vi "Create HDF5 chunked dataset (1D).vi"(5 "block size":i32, 6 "compression":i32, 8 "error in (no error)":errorcluster, 9 "data type":variant, 10 "name":string="stuff", 11 "ref in":T1 format="%.0x") -> (0 "error out":errorcluster, 3 "dset out":i32)   [LabVIEW 2013]
uses:
  <vilib>/addons/h5labview2/base/hid_t.ctl
  <vilib>/addons/h5labview2/dataset/H5D.lvlib
  <vilib>/addons/h5labview2/space/H5S.lvlib
  <vilib>/addons/h5labview2/props/H5P.lvlib
  <vilib>/addons/h5labview2/type/H5T.lvlib
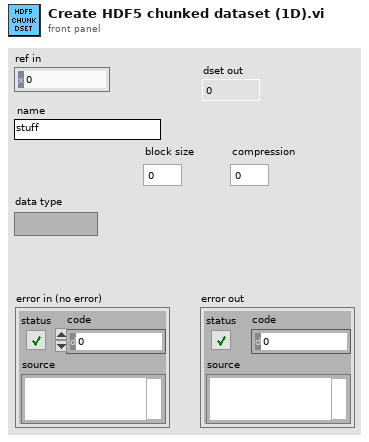
[diagram p1: front panel]
types:
  T1 = typedef "hid_t.ctl" = i32
  T2 = enum16{"H5P_ROOT", "H5P_OBJECT_CREATE", "H5P_FILE_CREATE", "H5P_FILE_ACCESS", "H5P_DATASET_CREATE", "H5P_DATASET_ACCESS", "H5P_DATASET_XFER", "H5P_FILE_MOUNT", "H5P_GROUP_CREATE", "H5P_GROUP_ACCESS", "H5P_DATATYPE_CREATE", "H5P_DATATYPE_ACCESS", "H5P_STRING_CREATE", "H5P_ATTRIBUTE_CREATE", "H5P_OBJECT_COPY", "H5P_LINK_CREATE", "H5P_LINK_ACCESS"}
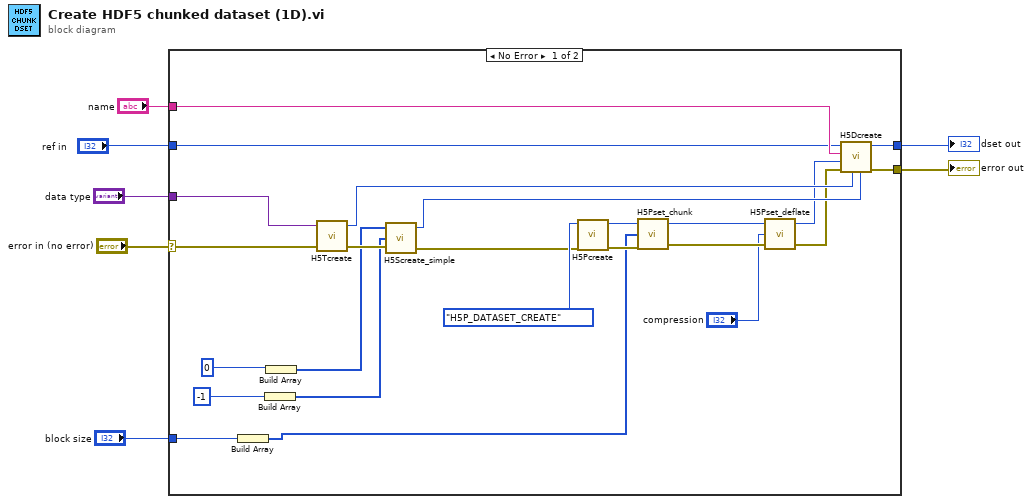
[diagram p0: block diagram]
diagram:
  n1 = case shown="No Error" "error in (no error)" {
    selector: "error in (no error)" -> [w12 w32]
    tunnel: [w31 w32] -> w7
    tunnel: [w30 _] -> w6
    tunnel: "name" -> [w24 _]
    tunnel: "ref in" -> [w23 _]
    tunnel: "data type" -> [w22 _]
    tunnel: "block size" -> [w21 _]
    frame No Error {
      n2 = Build Array(w21) -> (w20:i32[])
      n3 = Build Array(-1 ("element")) -> (w8:i32[])
      n4 = Build Array(0 ("element")) -> (w10:i32[])
      n5 = call <vilib>:"H5Tcreate.vi"("error in (no error)"=w12, "type variant"=w22) -> ("error out"=w19:errorcluster, "type out"=w28:i32)  [unwired: 2 in]
      n6 = call <vilib>:"H5Screate_simple.vi"("error in (no error)"=w19, "maxdims"=w8, "dims"=w10) -> ("error out"=w18:errorcluster, "space out"=w29:T1)  [unwired: 1 out]
      n7 = call <vilib>:"H5Pcreate.vi"("error in (no error)"=w18, "prop class (DATASET_CREATE)"=T2."H5P_DATASET_CREATE" ("prop class")) -> ("error out"=w26:errorcluster, "ref out"=w27:T1)  [unwired: 4 in]
      n8 = call <vilib>:"H5Pset_chunk.vi"("error in (no error)"=w26, "chunk size"=w20, "prop in"=w27) -> ("error out"=w16:errorcluster, "prop out"=w17:T1)  [unwired: 1 in]
      n9 = call <vilib>:"H5Pset_deflate.vi"("error in (no error)"=w16, "level"="compression", "prop in"=w17) -> ("error out"=w13:errorcluster, "prop out"=w14:T1)  [unwired: 1 in]
      n10 = call <vilib>:"H5Dcreate.vi"("space id"=w29, "type id"=w28, "error in (no error)"=w13, "props id"=w14, "name"=w24, "loc in"=w23) -> ("error out"=w31:errorcluster, "dset out"=w30:T1)  [unwired: 2 in]
    }
    frame Error {
    }
  }
  "error out" <- w7
  "dset out" <- w6
